vi "globalStartAuto.vi"() -> ()   [LabVIEW 2017]
uses:
  controls/gcodeArray.ctl
panel:
  out "G-Code Array 2":T1=["Loi khong ket noChua Chon File"]
  in  "Start Auto":bool
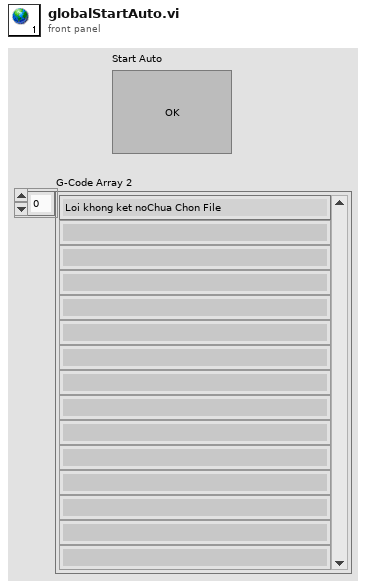
[diagram p1: front panel]
types:
  T1 = typedef "gcodeArray.ctl" = string[]
diagram:
